vi "ReadScan_Rf2.vi"(8 "error in (no error)":errorcluster, 11 "Data In":T3) -> (0 "error out":errorcluster, 1 "Next State":T2=enum."State1", 2 "States":T1, 3 "Data Out":T3)   [LabVIEW 2014]
doc: "Use this template to build a standard state machine design pattern. Each state executes code and determines which state to transition to. Contrast this design pattern with the User Interface Event Handler pattern, in which code executes in response to user actions. Contrast this design pattern also with the Queued Message Handler pattern, in which each message handling code can queue zero or more new messages.\nNote: This template does not contain the most recent programming guidelines recommended by National Instruments. For a complete, project-based implementation of the Standard State Machine pattern, use the Create Project dialog box instead of this template."
uses:
  controls/Data.ctl
  controls/Wait Scan States.ctl
  controls/State.ctl
  controls/ReadScan1States.ctl
panel:
  # "日期"
  # "機種名稱"
  # "機種代號"
  # "商品條碼"
  # "台"
  # "OK"
  # "NG"
  # "台"
  # "總計"
  # "台"
  # "日期"
  # "機種名稱"
  # "機種代號"
  # "商品條碼"
  # "台"
  # "OK"
  # "NG"
  # "台"
  # "總計"
  # "台"
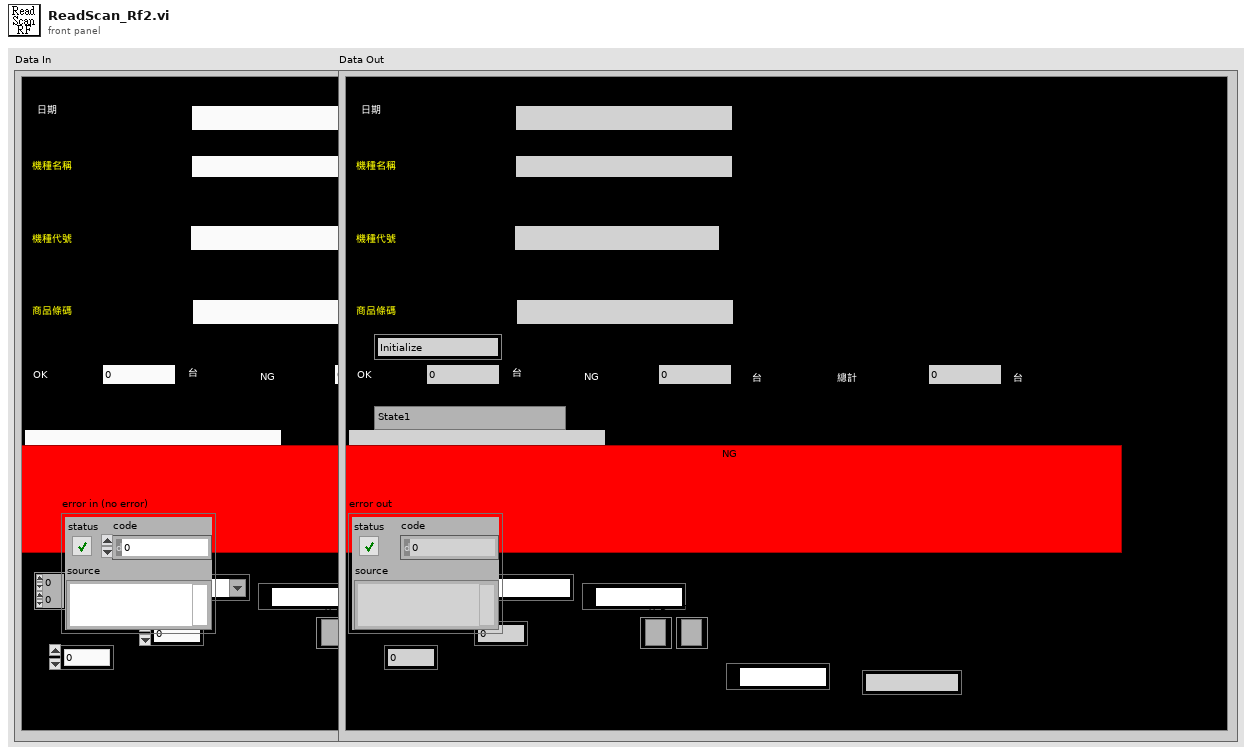
[diagram p1: front panel]
types:
  T1 = typedef "State.ctl" = enum16{"Initialize", "Wait for Scan", "State 1", "State 2", "NG", "NG1", "OK", "OKNG", "OKNG1", "Exit"}
  T2 = typedef "Wait Scan States.ctl" = enum16{"Initialize", "State1", "Stop"}
  T3 = typedef "Data.ctl" = cluster{"Date":string, "BarCode1":string, "BarCode2":string, "BarCode3":string, "Message":string, "OK Count":u16, "NG Count":u16, "Total Count":u16, "ModelData":string[][], "OK&NG":bool, "COM1":refnum<visa-resource-name>, "COM2":refnum<visa-resource-name>, "IO":i32, "Time":u32, "TCP":refnum<k5>, "TCP 2":refnum<k5>, "COM3":refnum<visa-resource-name>, "CheckPars":string}
  T4 = typedef "ReadScan1States.ctl" = enum16{"Initialize", "Init2", "Step1", "Step2", "Step3", "Step4", "One", "Two", "Three", "Four", "Five", "End", "Stop"}
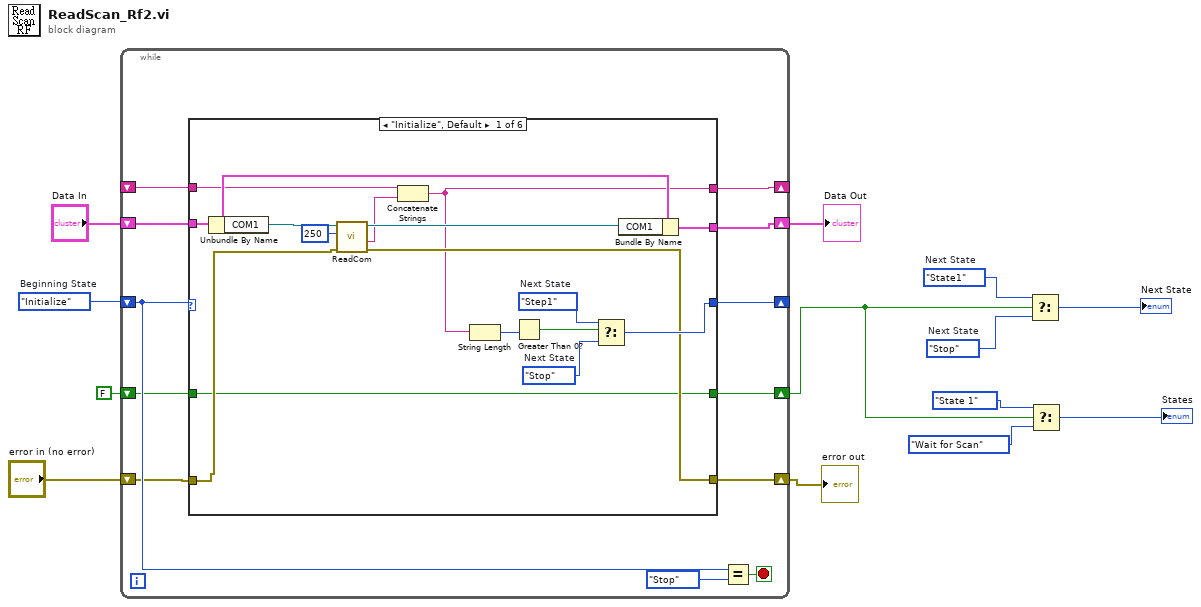
[diagram p0: block diagram]
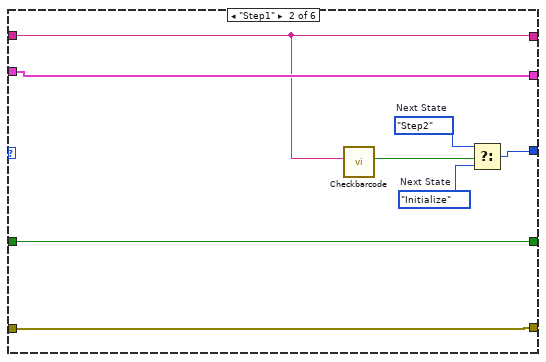
[diagram p2: hidden frame]
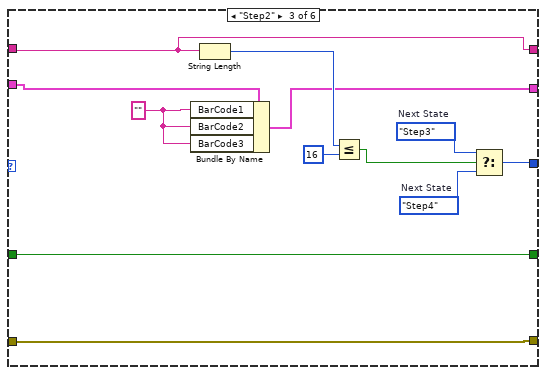
[diagram p3: hidden frame]
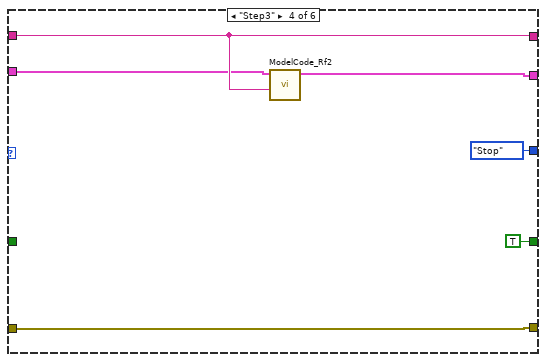
[diagram p4: hidden frame]
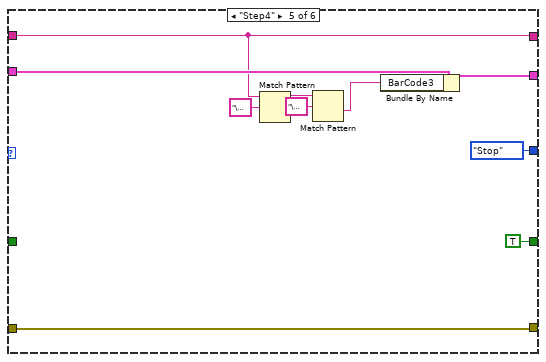
[diagram p5: hidden frame]
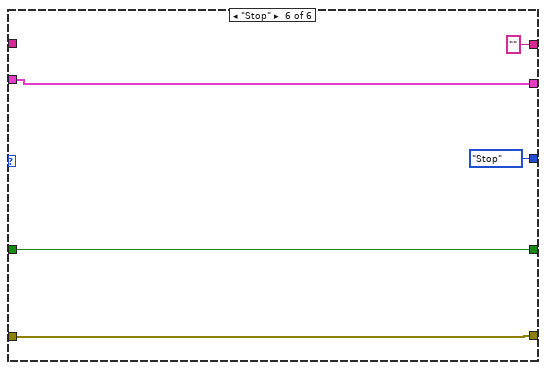
[diagram p6: hidden frame]
diagram:
  w8 = Wait_Scan_States."State1"  # Next State
  w7 = Wait_Scan_States."Stop"  # Next State
  w13 = ReadScan1States."Initialize"  # Beginning State
  n1 = while {
    shift-right: [w22] -> _
    shift-left: w13 -> [w23]
    shift-right: [w17] -> w11
    shift-left: "Data In" -> [w20]
    shift-right: [w16] -> w9
    shift-left: "error in (no error)" -> [w21]
    shift-right: [w18] -> _
    shift-left: _ -> [w19]
    shift-right: [w15] -> w1
    shift-left: FALSE -> [w14]
    stop <- w25 stop-if-true
    n2 = case shown="\"Initialize\", Default" w23 {
      tunnel: [w36 w46 w56 ReadScan1States."Stop" ("Next State") ReadScan1States."Stop" ("Next State") ReadScan1States."Stop" ("Next State")] -> w22
      tunnel: w21 -> [w32 w44 w54 w67 w76 w79]
      tunnel: w20 -> [w35 w49 w52 w64 w75 w80]
      tunnel: w19 -> [w29 w43 w55 w65 w73 _]
      tunnel: [w26 w43 w55 w65 w73 ""] -> w18
      tunnel: [w34 w49 w51 w63 w74 w80] -> w17
      tunnel: [w31 w44 w54 w67 w76 w79] -> w16
      tunnel: [w30 w45 w53 TRUE TRUE w78] -> w15
      tunnel: w14 -> [w30 w45 w53 _ _ w78]
      frame "Initialize", Default {
        w38 = ReadScan1States."Step1"  # Next State
        w37 = ReadScan1States."Stop"  # Next State
        n3 = Unbundle By Name(w35) -> ("COM1"=w41:refnum<visa-resource-name>)
        n4 = call "ReadCom.vi"("error in (no error)"=w32, "delay before read (ms)"=u32 250, "Com In"=w41) -> ("error out"=w31:errorcluster, "Response"=w28:string, "Com Out"=w33:refnum<visa-resource-name>)  [unwired: 5 in, 1 out]
        n5 = Concatenate Strings(w29, w28) -> (w26:string)
        n6 = String Length(string=w26) -> (length=w27:i32)
        n7 = Greater Than 0?(x=w27) -> (x > 0?=w39:bool)
        n8 = Select(t=w38, s=w39, f=w37) -> (s? t:f=w36:T4)
        n9 = Bundle By Name(cluster=w35, "COM1"=w33) -> (w34:T3)
      }
      frame "Step1" {
        w48 = ReadScan1States."Step2"  # Next State
        w47 = ReadScan1States."Initialize"  # Next State
        n10 = call "Checkbarcode.vi"("String In"=w43) -> ("Complete"=w42:bool)  [unwired: 10 in]
        n11 = Select(t=w48, s=w42, f=w47) -> (s? t:f=w46:T4)
      }
      frame "Step2" {
        w50 = "" ("BarCode1")
        w59 = ReadScan1States."Step3"  # Next State
        w58 = ReadScan1States."Step4"  # Next State
        n12 = Bundle By Name(cluster=w52, "BarCode1"=w50, "BarCode2"=w50, "BarCode3"=w50) -> (w51:T3)
        n13 = String Length(string=w55) -> (length=w61:i32)
        n14 = Less Or Equal?(x=w61, y=16) -> (x <= y?=w57:bool)
        n15 = Select(t=w59, s=w57, f=w58) -> (s? t:f=w56:T4)
      }
      frame "Step3" {
        n16 = call "ModelCode_Rf2.vi"("BarCode"=w65, "Data In"=w64) -> ("Data Out"=w63:T3)  [unwired: 8 in, 1 out]
      }
      frame "Step4" {
        n17 = Match Pattern(string=w73, regular expression="\u0003") -> (before substring=w71:string)  [unwired: 1 in, 3 out]
        n18 = Match Pattern(string=w71, regular expression="\u0002") -> (after substring=w69:string)  [unwired: 1 in, 3 out]
        n19 = Bundle By Name(cluster=w75, "BarCode3"=w69) -> (w74:T3)
      }
      frame "Stop" {
      }
    }
    n20 = Equal?(x=w23, y=ReadScan1States."Stop" ("States")) -> (x = y?=w25:bool)
  }
  "Data Out" <- w11
  "error out" <- w9
  n21 = Select(t=w8, s=w1, f=w7) -> (s? t:f=→"Next State":T2)
  n22 = Select(t=State."State 1" ("States"), s=w1, f=State."Wait for Scan" ("States")) -> (s? t:f=→"States":T1)
